vi "simple_camera_control.vi"(7 "Sensitivity":dbl=1000.0, 8 "Y":dbl, 9 "X":dbl, 10 "Window":refnum<vi>, 11 "Display":refnum<vi>) -> ()   [LabVIEW 2009]
uses:
  <vilib>/Utility/miscctls.llb/LV3DPointTypeDef.ctl
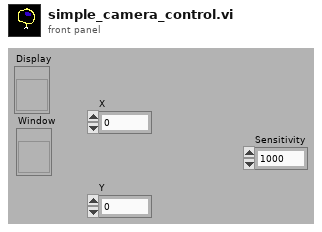
[diagram p1: front panel]
types:
  T1 = typedef "LV3DPointTypeDef.ctl" = cluster{"X":sgl, "Y":sgl, "Z":sgl}
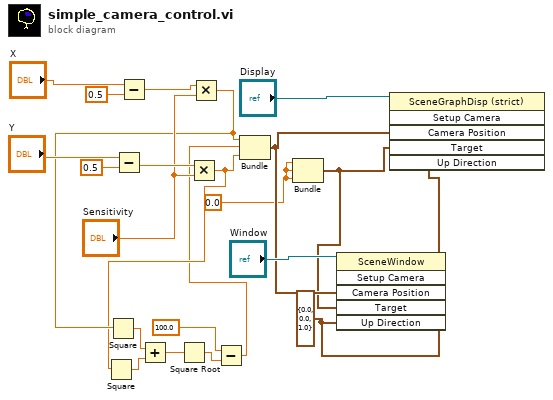
[diagram p0: block diagram]
diagram:
  w9 = 0.0 ("y")
  w11 = T1 {"X"=0.0, "Y"=0.0, "Z"=1.0} ("Up Direction")
  n1 = Subtract(x="Y", y=0.5) -> (x-y=w17:dbl)
  n2 = Subtract(x="X", y=0.5) -> (x-y=w16:dbl)
  n3 = Multiply(x=w17, y="Sensitivity") -> (x*y=w3:dbl)
  n4 = Square(x=w3) -> (x^2=w5:dbl)
  n5 = Multiply(x=w16, y="Sensitivity") -> (x*y=w4:dbl)
  n6 = Square(x=w4) -> (x^2=w6:dbl)
  n7 = Add(x=w6, y=w5) -> (x+y=w7:dbl)
  n8 = Square Root(x=w7) -> (sqrt(x)=w8:dbl)
  n9 = Subtract(x=100.0 ("y"), y=w8) -> (x-y=w1:dbl)
  n10 = Bundle(w4, w1, w3) -> (w12:cluster{dbl, dbl, dbl})  [unwired: 1 in]
  n11 = Bundle("y"=w9, "y"=w9, "y"=w9) -> (w10:cluster{"y":dbl, "y":dbl, "y":dbl})  [unwired: 1 in]
  n12 = invoke class="SceneWindow" method="Setup Camera"(reference="Window", "Camera Position"=w12, "Target"=w10, "Up Direction"=w11) -> ()  [unwired: 2 in, 6 out]
  n13 = invoke on="Invoke Node" class="SceneGraphDisp (strict)" method="Setup Camera"(reference="Display", "Camera Position"=w12, "Target"=w10, "Up Direction"=w11) -> ()  [unwired: 2 in, 6 out]
